vi "Get Tau.vi"(6 "ErrorCallOn":bool, 7 "init":bool=TRUE, 9 "CalType":enum8{"DFT-1", "DFT-5", "LRS"}(ring)=enum."LRS", 10 "Dt":dbl, 11 "X":dbl[](array[numeric])) -> (0 "B":dbl, 1 "A":dbl, 2 "e_tau":dbl, 3 "tau":dbl)   [LabVIEW 2015, in "Math Utilities.lvlib"]
doc: "This VI uses the techniques in Everest and Atkinson [2008] to determine the decay time constant of an exponential function with no background subtraction required. There are three techniques coded with one technique (LRS) coded in both Labview and C (and compiled in a dll). According to Everest and Atkinson, the DFT routines should be on par in terms of computation time with that of the LRS while the LRS should be substantially less susceptible to noise. According to the authors, the LRS and DFT routines should proceed in about 200 us for a 1000 point data sets. A description of the techniques is given in the block diagram.\n\n1. Initialize the VI so that we only have to do certain calculations required by the routine one time. For the DFT routines, we will calculate the sine and cosine of the angular frequency (wk = 2*pi*k/(N*dt)) as well as the weights used in the DFT-5 calculation. Since the average is weighted, the average of the tau's given by each of the frequency components will be sum(w_k*tau_k)/sum(w_k) where the values are summed over 1...5. For the LRS routines, the sums over t and t^2 can be determined apriori and therefore we only need to do them when we initialize. Bundle all of these into a single cluster and pick off the values required by the different routines.\n\n2. Solve for tau using one of the routines given in Everest and Atkinson [2008]. The DFT routines are fast on both a dual core and quad core machine (on the order of 10s of microseconds) while the LRS routines both incur substantial penalties for the explicit integration (1.5 ms for the Labview based solution and 750 us for the dll based routine. The DFT-5 is less susceptible to noise than the DFT-1 while the LRS routine is significantly better at noise rejection than the DFT."
uses:
  Math Utilities.lvlib
  <vilib>/Analysis/baseanly.llb/Matrix Type of Inverse Matrix.ctl
  <vilib>/Analysis/2dsp.llb/Real FFT.vi
  <vilib>/Analysis/7linalg.llb/Solve Linear Equations (single right hand).vi
  <vilib>/Analysis/baseanly.llb/Solve Linear Equations By Cholesky.vi
  <vilib>/Analysis/baseanly.llb/Real Matrix to Compact Array.vi
  <vilib>/Analysis/baseanly.llb/Real Compact Tri-Matrix Linear Eqs.vi
  <vilib>/Analysis/7linalg.llb/Solve Linear Eqs (General).vi
  <vilib>/Analysis/7linalg.llb/Solve Linear Eqs (Gen, single right hand).vi
  <vilib>/Analysis/Matrix/Numeric/Conversions/Array To Matrix - RA2.vi
  <vilib>/Analysis/NI_AALPro.lvlib
  <vilib>/Analysis/NI_AALBase.lvlib
  <vilib>/Analysis/Matrix/NI_Matrix.lvlib
panel:
  in  "error in":errorcluster
  out "error out":errorcluster
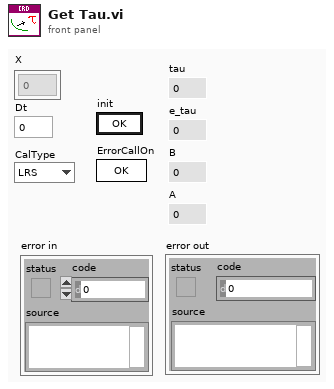
[diagram p1: front panel]
types:
  T1 = typedef "NI_AALBase.lvlib/Matrix Type of Inverse Matrix.ctl" = enum32{"General", "Positive Definite", "Lower Triangular", "Upper Triangular"}
  T2 = cluster{"NumSamp":i32, dbl[], dbl[], dbl[], dbl, "Ramp":dbl[], "St":dbl, "Stt":dbl}
  T3 = typedef "NI_Matrix.lvlib/RealMatrix.ctl" = dbl[][]
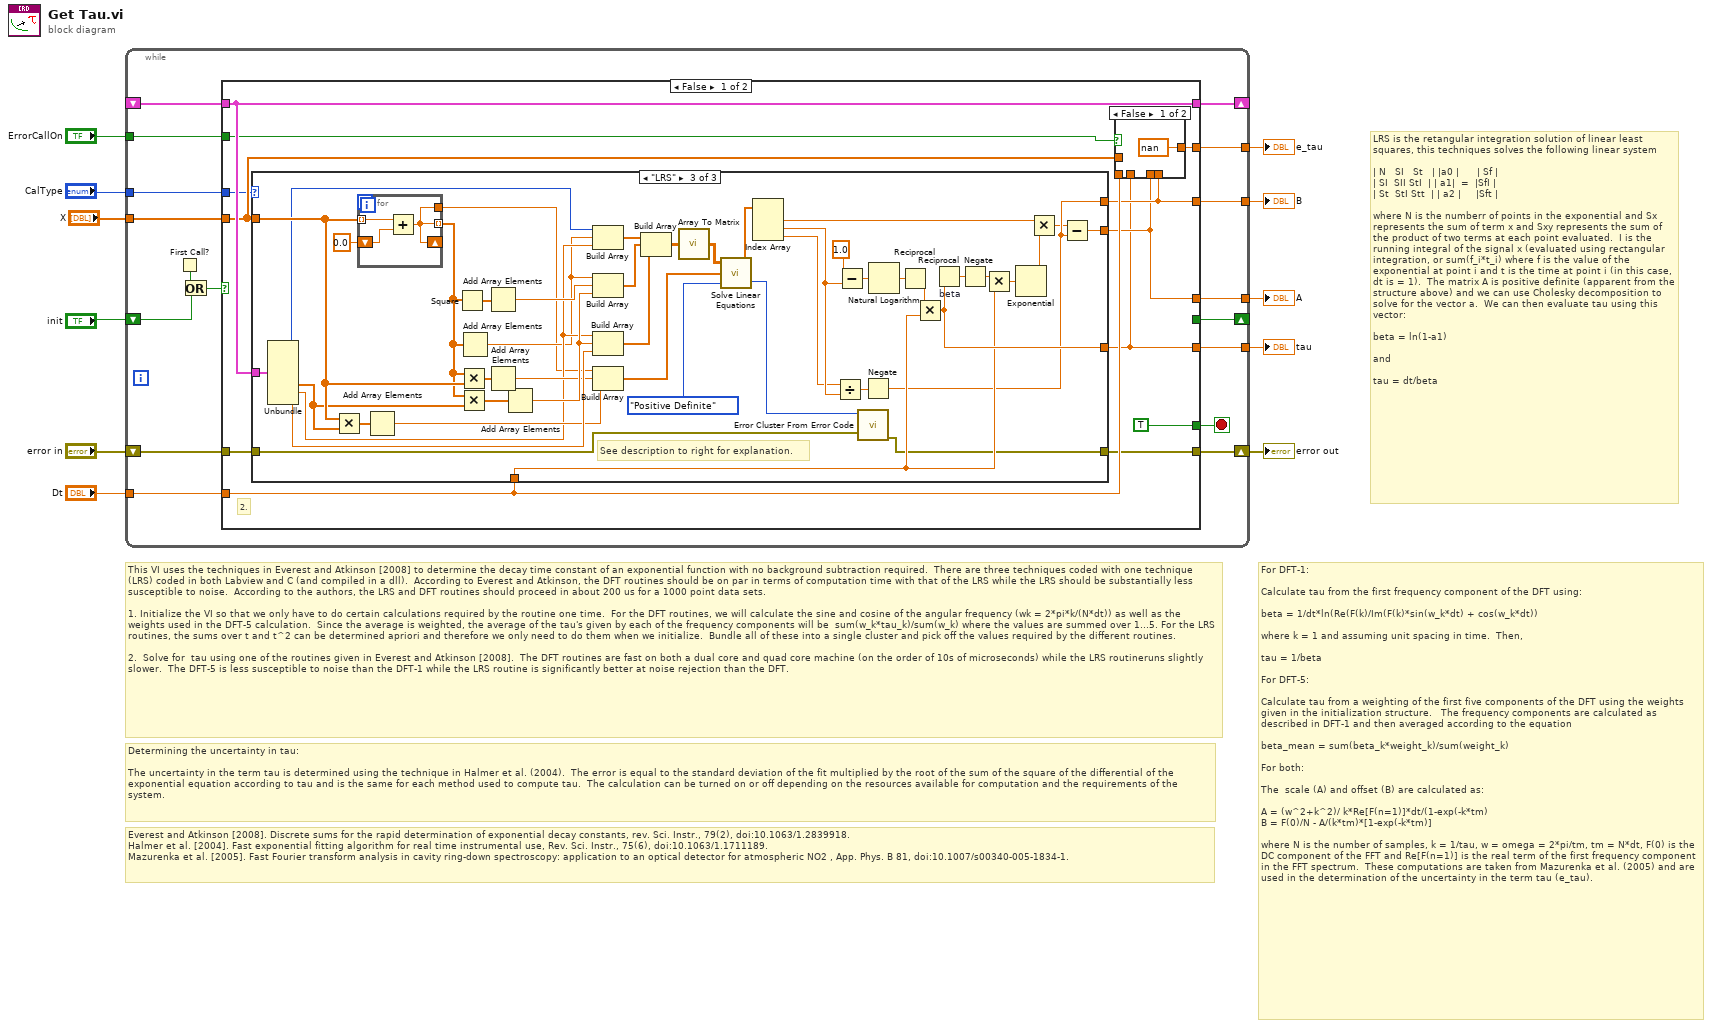
[diagram p0: block diagram]
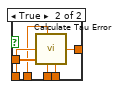
[diagram p2: hidden frame]
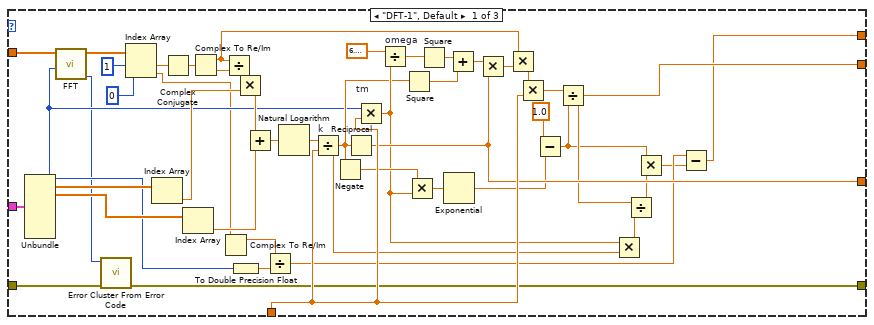
[diagram p3: hidden frame]
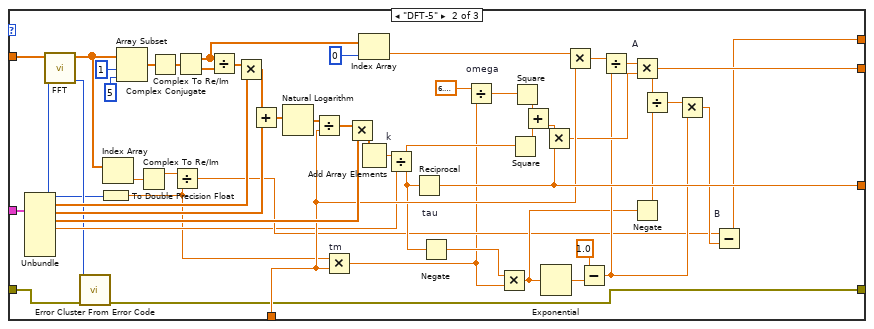
[diagram p4: hidden frame]
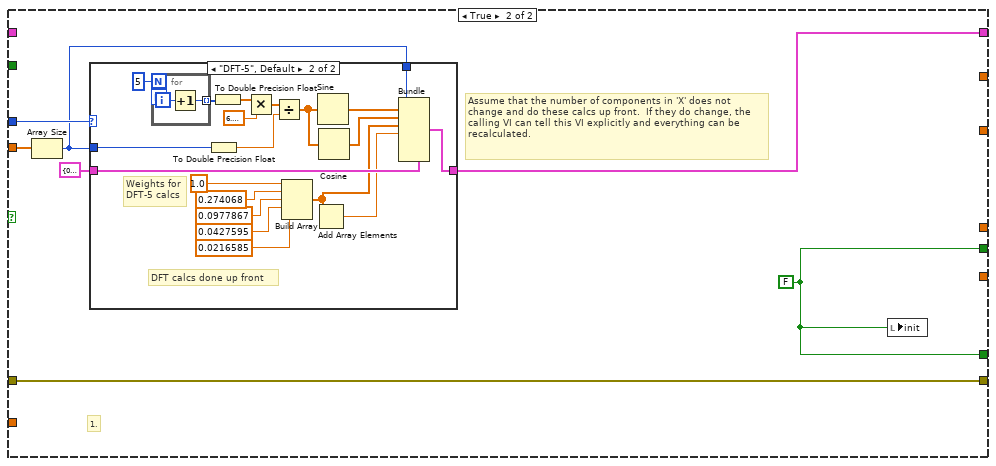
[diagram p5: hidden frame]
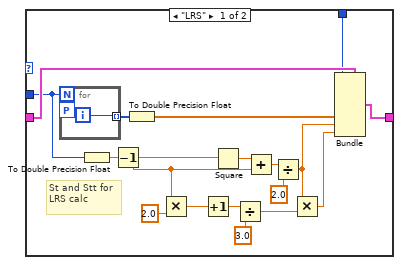
[diagram p6: hidden frame]
diagram:
  # "Determining the uncertainty in tau:\n \nThe uncertainty in the term tau is determined using the technique in Halmer et al. (2004).  The error is equal to the standard deviation of the fit multiplied by the root of the sum of the square of the differential of the exponential equation according to tau and is the same for each method used to compute tau.  The calculation can be turned on or off depending on the resources available for computation and the requirements of the system."
  # "For DFT-1:\n\nCalculate tau from the first frequency component of the DFT using:\n\nbeta = 1/dt*ln(Re(F(k)/Im(F(k)*sin(w_k*dt) + cos(w_k*dt))\n\nwhere k = 1 and assuming unit spacing in time.  Then, \n\ntau = 1/beta\n\nFor DFT-5:\n\nCalculate tau from a weighting of the first five components of the DFT using the weights given in the initialization structure.   The frequency components are calculated as described in DFT-1 and then averaged according to the equation\n\nbeta_mean = sum(beta_k*weight_k)/sum(weight_k)\n\nFor both:\n\nThe  scale (A) and offset (B) are calculated as:\n\nA = (w^2+k^2)/ k*Re[F(n=1)]*dt/(1-exp(-k*tm)\nB = F(0)/N - A/(k*tm)*[1-exp(-k*tm)]\n\nwhere N is the number of samples, k = 1/tau, w = omega = 2*pi/tm, tm = N*dt, F(0) is the DC component of the FFT and Re[F(n=1)] is the real term of the first frequency component in the FFT spectrum.  These computations are taken from Mazurenka et al. (2005) and are used in the determination of the uncertainty in the term tau (e_tau)."
  # "Everest and Atkinson [2008]. Discrete sums for the rapid determination of exponential decay constants, rev. Sci. Instr., 79(2), doi:10.1063/1.2839918.\nHalmer et al. [2004]. Fast exponential fitting algorithm for real time instrumental use, Rev. Sci. Instr., 75(6), doi:10.1063/1.1711189.\nMazurenka et al. [2005]. Fast Fourier transform analysis in cavity ring-down spectroscopy: application to an optical detector for atmospheric NO2 , App. Phys. B 81, doi:10.1007/s00340-005-1834-1."
  # "LRS is the retangular integration solution of linear least squares, this techniques solves the following linear system \n\n| N   SI   St   | |a0 |      | Sf |\n| SI  SII StI  | | a1|  =  |SfI |\n| St  StI Stt  | | a2 |     |Sft |\n\nwhere N is the numberr of points in the exponential and Sx represents the sum of term x and Sxy represents the sum of the product of two terms at each point evaluated.  I is the running integral of the signal x (evaluated using rectangular integration, or sum(f_i*t_i) where f is the value of the exponential at point i and t is the time at point i (in this case, dt is = 1).  The matrix A is positive definite (apparent from the structure above) and we can use Cholesky decomposition to solve for the vector a.  We can then evaluate tau using this vector:\n\nbeta = ln(1-a1)\n\nand \n\ntau = dt/beta"
  # "This VI uses the techniques in Everest and Atkinson [2008] to determine the decay time constant of an exponential function with no background subtraction required.  There are three techniques coded with one technique (LRS) coded in both Labview and C (and compiled in a dll).  According to Everest and Atkinson, the DFT routines should be on par in terms of computation time with that of the LRS while the LRS should be substantially less susceptible to noise.  According to the authors, the LRS and DFT routines should proceed in about 200 us for a 1000 point data sets. \n\n1. Initialize the VI so that we only have to do certain calculations required by the routine one time.  For the DFT routines, we will calculate the sine and cosine of the angular frequency (wk = 2*pi*k/(N*dt)) as well as the weights used in the DFT-5 calculation.  Since the average is weighted, the average of the tau's given by each of the frequency components will be  sum(w_k*tau_k)/sum(w_k) where the values are summed over 1...5. For the LRS routines, the sums over t and t^2 can be determined apriori and therefore we only need to do them when we initialize.  Bundle all of these into a single cluster and pick off the values required by the different routines.\n\n2.  Solve for  tau using one of the routines given in Everest and Atkinson [2008].  The DFT routines are fast on both a dual core and quad core machine (on the order of 10s of microseconds) while the LRS routineruns slightly slower.  The DFT-5 is less susceptible to noise than the DFT-1 while the LRS routine is significantly better at noise rejection than the DFT."
  n1 = while {
    shift-right: [w25] -> _
    shift-left: _ -> [w28]
    tunnel: "Dt" -> [w23]
    tunnel: "ErrorCallOn" -> [w21]
    tunnel: "X" -> [w20]
    tunnel: [w19] -> w7
    tunnel: [w18] -> w6
    tunnel: [w17] -> w5
    tunnel: [w16] -> w4
    tunnel: "CalType" -> [w13]
    shift-right: [w15] -> w3
    shift-left: "error in" -> [w14]
    shift-right: [w12] -> _
    shift-left: "init" -> [w22]
    stop <- w24 stop-if-true
    n2 = First Call?() -> (First Call?: T/F=w26:bool)
    n3 = Or(x=w26, y=w22) -> (x .or. y?=w27:bool)
    n4 = case shown="False" w27 {
      tunnel: w20 -> [w39 w202]
      tunnel: [w40 w198] -> w25
      tunnel: w28 -> [w40 _]
      tunnel: [TRUE w197] -> w24
      tunnel: w23 -> [w37 _]
      tunnel: w21 -> [w29 _]
      tunnel: [w36 _] -> w19
      tunnel: [w35 _] -> w18
      tunnel: [w34 _] -> w17
      tunnel: [w33 _] -> w16
      tunnel: [w32 w201] -> w15
      tunnel: w14 -> [w31 w201]
      tunnel: w13 -> [w30 w200]
      tunnel: [_ w197] -> w12
      frame False {
        # "2."
        n5 = case shown="\"LRS\"" w30 {
          tunnel: w39 -> [w80 w136 w191]
          tunnel: w40 -> [w89 w135 w192]
          tunnel: w37 -> [w71 w125 w189]
          tunnel: [w69 w128 w190] -> w33
          tunnel: [w62 w114 w188] -> w34
          tunnel: [w57 w107 w187] -> w35
          tunnel: [w48 w97 w152] -> w32
          tunnel: w31 -> [w50 w98 w151]
          frame "DFT-1", Default {
            n6 = Unbundle(w89) -> ("NumSamp"=w54:i32, w88:dbl[], w87:dbl[])  [unwired: 5 out]
            n7 = call-poly <vilib>:"FFT.vi"("FFT size"=w54, "X"=w80) -> ("error"=w49:i32, "FFT {X}"=w84:cdb[])  [unwired: 1 in, 7 out]
            n8 = call <vilib>:"Error Cluster From Error Code.vi"("error in (no error)"=w50, "error code (0)"=w49) -> ("error out"=w48:errorcluster)  [unwired: 7 in]
            n9 = Index Array(array=w84, index #1=1 ("index"), index #2=0 ("index")) -> (element #1=w82:cdb, element #2=w52:cdb)
            n10 = Index Array(array=w88) -> (element=w86:dbl)  [unwired: 1 in]
            n11 = Complex Conjugate(1:w82) -> (0:w90:cdb)
            n12 = Index Array(array=w87) -> (element=w85:dbl)  [unwired: 1 in]
            n13 = Complex To Re/Im(x + iy=w90) -> (x=w74:dbl, y=w91:dbl)
            n14 = Complex To Re/Im(x + iy=w52) -> (x=w51:dbl)  [unwired: 1 out]
            n15 = Divide(x=w74, y=w91) -> (x/y=w94:dbl)
            n16 = To Double Precision Float(number=w54) -> (double precision float=w53:dbl)
            n17 = Multiply(x=w94, y=w86) -> (x*y=w93:dbl)
            n18 = Add(x=w93, y=w85) -> (x+y=w92:dbl)
            n19 = Divide(x=w51, y=w53) -> (x/y=w63:dbl)
            n20 = Natural Logarithm(1:w92) -> (0:w81:dbl)
            n21 = Divide "k"(x=w81, y=w71) -> (x/y=w55:dbl)
            n22 = Negate(x=w55) -> (-x=w68:dbl)
            n23 = Reciprocal(x=w55) -> (1/x=w69:dbl)
            n24 = Multiply "tm"(x=w54, y=w71) -> (x*y=w56:dbl)
            n25 = Divide "omega"(x=6.283185307179586, y=w56) -> (x/y=w78:dbl)
            n26 = Square(x=w55) -> (x^2=w77:dbl)
            n27 = Multiply(x=w68, y=w56) -> (x*y=w67:dbl)
            n28 = Square(x=w78) -> (x^2=w76:dbl)
            n29 = Exponential(1:w67) -> (0:w66:dbl)
            n30 = Add(x=w76, y=w77) -> (x+y=w75:dbl)
            n31 = Multiply(x=w75, y=w69) -> (x*y=w73:dbl)
            n32 = Multiply(x=w74, y=w73) -> (x*y=w72:dbl)
            n33 = Multiply(x=w72, y=w71) -> (x*y=w65:dbl)
            n34 = Subtract(x=1.0, y=w66) -> (x-y=w60:dbl)
            n35 = Divide ("A")(x=w65, y=w60) -> (x/y=w62:dbl)
            n36 = Multiply(x=w56, y=w55) -> (x*y=w61:dbl)
            n37 = Divide(x=w62, y=w61) -> (x/y=w59:dbl)
            n38 = Multiply(x=w60, y=w59) -> (x*y=w58:dbl)
            n39 = Subtract ("B")(x=w63, y=w58) -> (x-y=w57:dbl)
          }
          frame "DFT-5" {
            n40 = Unbundle(w135) -> ("NumSamp"=w96:i32, w134:dbl[], w133:dbl[], w126:dbl[], w103:dbl)  [unwired: 3 out]
            n41 = call-poly <vilib>:"FFT.vi"("FFT size"=w96, "X"=w136) -> ("error"=w99:i32, "FFT {X}"=w111:cdb[])  [unwired: 1 in, 7 out]
            n42 = call <vilib>:"Error Cluster From Error Code.vi"("error in (no error)"=w98, "error code (0)"=w99) -> ("error out"=w97:errorcluster)  [unwired: 7 in]
            n43 = To Double Precision Float(number=w96) -> (double precision float=w95:dbl)
            n44 = Index Array(array=w111) -> (element=w110:cdb)  [unwired: 1 in]
            n45 = Array Subset(array=w111, index=1, length=5) -> (w141:cdb[])
            n46 = Complex To Re/Im(x + iy=w110) -> (x=w109:dbl)  [unwired: 1 out]
            n47 = Complex Conjugate(1:w141) -> (0:w139:cdb[])
            n48 = Divide(x=w109, y=w95) -> (x/y=w108:dbl)
            n49 = Complex To Re/Im(x + iy=w139) -> (x=w102:dbl[], y=w140:dbl[])
            n50 = Divide(x=w102, y=w140) -> (x/y=w127:dbl[])
            n51 = Multiply(x=w127, y=w134) -> (x*y=w144:dbl[])
            n52 = Add(x=w144, y=w133) -> (x+y=w143:dbl[])
            n53 = Natural Logarithm(1:w143) -> (0:w142:dbl[])
            n54 = Divide(x=w142, y=w125) -> (x/y=w132:dbl[])
            n55 = Multiply "tm"(x=w95, y=w125) -> (x*y=w106:dbl)
            n56 = Multiply(x=w132, y=w126) -> (x*y=w138:dbl[])
            n57 = Index Array(array=w102, index=0) -> (element=w101:dbl)
            n58 = Add Array Elements(numeric array=w138) -> (sum=w137:dbl)
            n59 = Divide "k"(x=w137, y=w103) -> (x/y=w124:dbl)
            n60 = Reciprocal "tau"(x=w124) -> (1/x=w128:dbl)
            n61 = Negate(x=w124) -> (-x=w123:dbl)
            n62 = Divide "omega"(x=6.283185307179586, y=w106) -> (x/y=w104:dbl)
            n63 = Multiply(x=w123, y=w106) -> (x*y=w116:dbl)
            n64 = Square(x=w124) -> (x^2=w131:dbl)
            n65 = Square(x=w104) -> (x^2=w130:dbl)
            n66 = Add(x=w130, y=w131) -> (x+y=w129:dbl)
            n67 = Exponential(1:w116) -> (0:w122:dbl)
            n68 = Multiply(x=w129, y=w128) -> (x*y=w119:dbl)
            n69 = Multiply(x=w101, y=w125) -> (x*y=w120:dbl)
            n70 = Subtract(x=1.0, y=w122) -> (x-y=w117:dbl)
            n71 = Divide(x=w120, y=w117) -> (x/y=w118:dbl)
            n72 = Multiply "A"(x=w118, y=w119) -> (x*y=w114:dbl)
            n73 = Negate(x=w116) -> (-x=w115:dbl)
            n74 = Divide(x=w114, y=w115) -> (x/y=w113:dbl)
            n75 = Multiply(x=w113, y=w117) -> (x*y=w112:dbl)
            n76 = Subtract "B"(x=w108, y=w112) -> (x-y=w107:dbl)
          }
          frame "LRS" {
            # "See description to right for explanation."
            n77 = Unbundle(w192) -> ("NumSamp"=w149:i32, "Ramp"=w182:dbl[], "St"=w167:dbl, "Stt"=w179:dbl)  [unwired: 4 out]
            n78 = Multiply(x=w191, y=w182) -> (x*y=w177:dbl[])
            n79 = for {
              tunnel: w191 -> [w195] mode=indexing
              tunnel: [w193] -> w150 mode=indexing
              shift-right: [w193] -> _
              shift-left: 0.0 -> [w194]
              tunnel: [w193] -> w148
              n80 = Add(x=w195, y=w194) -> (x+y=w193:dbl)
            }
            n81 = Add Array Elements ("Sft")(numeric array=w177) -> (sum=w176:dbl)
            n82 = Square(x=w150) -> (x^2=w185:dbl[])
            n83 = Multiply(x=w150, y=w191) -> (x*y=w184:dbl[])
            n84 = Multiply(x=w150, y=w182) -> (x*y=w183:dbl[])
            n85 = Add Array Elements ("SI")(numeric array=w150) -> (sum=w166:dbl)
            n86 = Add Array Elements ("SII")(numeric array=w185) -> (sum=w181:dbl)
            n87 = Add Array Elements ("SfI")(numeric array=w184) -> (sum=w178:dbl)
            n88 = Add Array Elements ("StI")(numeric array=w183) -> (sum=w180:dbl)
            n89 = Build Array(w149, w166, w167) -> (w174:dbl[])
            n90 = Build Array(w166, w181, w180) -> (w173:dbl[])
            n91 = Build Array(w167, w180, w179) -> (w172:dbl[])
            n92 = Build Array(w148, w178, w176) -> (w175:dbl[])
            n93 = Build Array(w174, w173, w172) -> (w171:dbl[][])
            n94 = call-poly <vilib>:"Array To Matrix.vi"("Real 2D Array"=w171) -> ("Real Matrix"=w147:T3)
            n95 = call-poly <vilib>:"Solve Linear Equations.vi"("matrix type"=Matrix_Type_of_Inverse_Matrix."Positive Definite", "Known Vector"=w175, "Input Matrix"=w147) -> ("error"=w153:i32, "Solution Vector"=w163:dbl[])
            n96 = Index Array(array=w163) -> (element #1=w154:dbl, element #2=w157:dbl, element #3=w156:dbl)  [unwired: 3 in]
            n97 = Divide(x=w156, y=w157) -> (x/y=w162:dbl)
            n98 = Subtract(x=1.0, y=w157) -> (x-y=w169:dbl)
            n99 = call <vilib>:"Error Cluster From Error Code.vi"("error in (no error)"=w151, "error code (0)"=w153) -> ("error out"=w152:errorcluster)  [unwired: 7 in]
            n100 = Negate(x=w162) -> (-x=w187:dbl)
            n101 = Natural Logarithm(1:w169) -> (0:w168:dbl)
            n102 = Reciprocal(x=w168) -> (1/x=w165:dbl)
            n103 = Multiply(x=w165, y=w189) -> (x*y=w190:dbl)
            n104 = Reciprocal "beta"(x=w190) -> (1/x=w161:dbl)
            n105 = Negate(x=w161) -> (-x=w160:dbl)
            n106 = Multiply(x=w160, y=w189) -> (x*y=w159:dbl)
            n107 = Exponential(1:w159) -> (0:w155:dbl)
            n108 = Multiply(x=w154, y=w155) -> (x*y=w158:dbl)
            n109 = Subtract(x=w158, y=w187) -> (x-y=w188:dbl)
          }
        }
        n110 = case shown="False" w29 {
          tunnel: w39 -> [_ w47]
          tunnel: w37 -> [_ w46]
          tunnel: [nan ("e_tau") w45] -> w36
          tunnel: w35 -> [_ w44]
          tunnel: w34 -> [_ w43]
          tunnel: w33 -> [_ w42]
          frame False {
          }
          frame True {
            n111 = call "Calculate Tau Error.vi"("tau"=w42, "Dt"=w46, "X"=w47, "A"=w43, "B"=w44) -> ("e_tau"=w45:dbl)  [unwired: 4 in]
          }
        }
      }
      frame True {
        w197 = FALSE
        # "1."
        # "Assume that the number of components in 'X' does not change and do these calcs up front.  If they do change, the calling VI can tell this VI explicitly and everything can be recalculated."
        n112 = Array Size(array=w202) -> (size(s)=w199:i32)
        n113 = case shown="\"DFT-5\", Default" w200 {
          tunnel: w199 -> [w207 w229]
          tunnel: T2 {"NumSamp"=0, [], [], [], 0.0, "Ramp"=[], "St"=0.0, "Stt"=0.0} ("output cluster") -> [w220 w228]
          tunnel: w199 -> [w218 w227]
          tunnel: [w219 w222] -> w198
          frame "LRS" {
            # "St and Stt for LRS calc"
            n114 = for {
              N: w207 -> [_]
              tunnel: [w221] -> w217 mode=indexing
              workers-P: _ -> [_]
              i -> [w221]
            }
            n115 = To Double Precision Float(number=w207) -> (double precision float=w215:dbl)
            n116 = Decrement(x=w215) -> (x-1=w214:dbl)
            n117 = To Double Precision Float(number=w217) -> (double precision float=w216:dbl[])
            n118 = Multiply(x=w214, y=2.0) -> (x*y=w212:dbl)
            n119 = Increment(x=w212) -> (x+1=w206:dbl)
            n120 = Square(x=w214) -> (x^2=w208:dbl)
            n121 = Divide(x=w206, y=3.0) -> (x/y=w204:dbl)
            n122 = Add(x=w208, y=w214) -> (x+y=w209:dbl)
            n123 = Divide(x=w209, y=2.0) -> (x/y=w205:dbl)
            n124 = Multiply(x=w205, y=w204) -> (x*y=w203:dbl)
            n125 = Bundle(cluster=w220, "NumSamp"=w218, "Ramp"=w216, "St"=w205, "Stt"=w203) -> (w219:T2)  [unwired: 4 out]
          }
          frame "DFT-5", Default {
            # "DFT calcs done up front"
            # "Weights for DFT-5 calcs"
            n126 = for {
              N: 5 -> [_]
              tunnel: [w242] -> w237 mode=indexing
              workers-P: _ -> [_]
              i -> [w243]
              n127 = Increment(x=w243) -> (x+1=w242:i32)
            }
            n128 = To Double Precision Float(number=w229) -> (double precision float=w230:dbl)
            n129 = To Double Precision Float(number=w237) -> (double precision float=w238:dbl[])
            n130 = Multiply(x=w238, y=6.283185307179586) -> (x*y=w239:dbl[])
            n131 = Divide(x=w239, y=w230) -> (x/y=w240:dbl[])
            n132 = Build Array(1.0, 0.274068, 0.0977867, 0.0427595, 0.0216585) -> (w224:dbl[])
            n133 = Add Array Elements(numeric array=w224) -> (sum=w223:dbl)
            n134 = Sine(x=w240) -> (sin(x)=w226:dbl[])
            n135 = Cosine(x=w240) -> (cos(x)=w225:dbl[])
            n136 = Bundle(cluster=w228, "NumSamp"=w227, w226, w225, w224, w223) -> (w222:T2)  [unwired: 3 out]
          }
        }
        n137 = local write "init"(w197) -> ()
      }
    }
  }
  "e_tau" <- w7
  "B" <- w6
  "A" <- w5
  "tau" <- w4
  "error out" <- w3
